vi "Get Serial Number by Position.vi"(10 "Position":u32, 11 "Application.lvclass":refnum<class "Application.lvclass">) -> (3 "Value":string)   [LabVIEW 2017, in "Application.lvlib" / "Application.lvclass"]
doc: "Returns the serial number for a given position."
uses:
  Application.lvclass
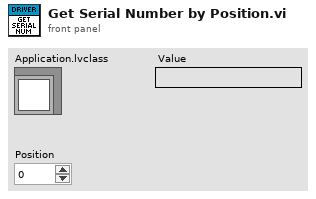
[diagram p1: front panel]
types:
  T1 = cluster{"Serial Number Reference":refnum<vi>, "Status Message Reference":refnum<vi>, "Position":u32}[]
  T2 = cluster{"Serial Number Reference":refnum<vi>, "Status Message Reference":refnum<vi>, "Position":u32}
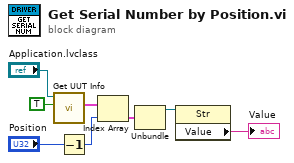
[diagram p0: block diagram]
diagram:
  n1 = call-dynamic "Get UUT Info.vi"("Scanned Only (false)"=TRUE, "Application in"="Application.lvclass") -> ("All UUTs"=w2:T1)  [unwired: 7 in, 2 out]
  n2 = Decrement(x="Position") -> (x-1=w5:u32)
  n3 = Index Array(array=w2, index=w5) -> (element=w6:T2)
  n4 = Unbundle(w6) -> ("Serial Number Reference"=w7:refnum<vi>)  [unwired: 2 out]
  n5 = property class="Str"(reference=w7) -> ("Value"=→"Value":string)  [unwired: 1 in, 2 out]
